vi "downsample 1D array - I16.vi"(2 "Ave N":dbl, 3 "Array In":i16[](array[numeric])) -> (1 "Array Out":i16[](array[numeric]))   [LabVIEW 2014]
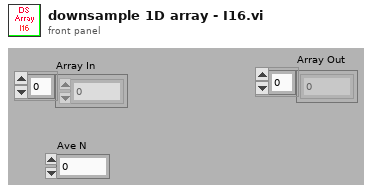
[diagram p1: front panel]
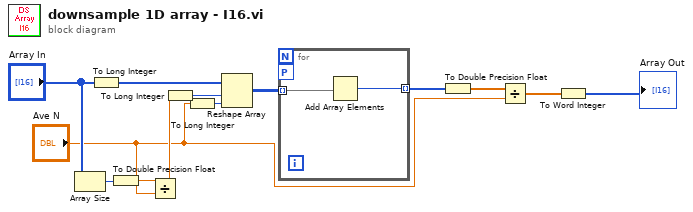
[diagram p0: block diagram]
diagram:
  n1 = Array Size(array="Array In") -> (size(s)=w12:i32)
  n2 = To Long Integer(number="Array In") -> (32bit integer=w8:i32[])
  n3 = To Double Precision Float(number=w12) -> (double precision float=w4:dbl)
  n4 = Divide(x=w4, y="Ave N") -> (x/y=w10:dbl)
  n5 = To Long Integer(number=w10) -> (32bit integer=w3:i32)
  n6 = To Long Integer(number="Ave N") -> (32bit integer=w2:i32)
  n7 = Reshape Array(w8, w3, w2) -> (w9:i32[][])
  n8 = for {
    tunnel: w9 -> [w15] mode=indexing
    tunnel: [w14] -> w11 mode=indexing
    workers-P: _ -> [_]
    n9 = Add Array Elements(numeric array=w15) -> (sum=w14:i32)
  }
  n10 = To Double Precision Float(number=w11) -> (double precision float=w1:dbl[])
  n11 = Divide(x=w1, y="Ave N") -> (x/y=w7:dbl[])
  n12 = To Word Integer(number=w7) -> (16bit integer=→"Array Out":i16[])
